vi "Pre Launch Init.vi"(11 "Child1 in":refnum<class "Child1.lvclass">) -> (0 "error out":errorcluster, 3 "Child1 out":refnum<class "Child1.lvclass">)   [LabVIEW 2020, in "Child1.lvclass"]
doc: "(<B>Filename</B>: Actor Framework.lvlib:Actor.lvclass:Pre Launch Init.vi)\n\nDefines behavior that occurs after the Launch Nested Actor method is invoked but before the actor's Actor Core method begins running.\n\nBy default, this method does nothing. A descendant class may override it to define behavior."
uses:
  Child1.lvclass
  Child1.lvclass/Child1.ctl
  <vilib>/ActorFramework/Actor/Actor.lvclass
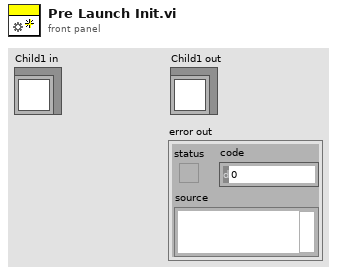
[diagram p1: front panel]
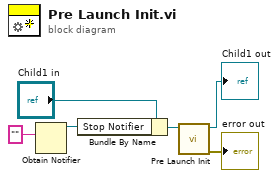
[diagram p0: block diagram]
diagram:
  n1 = Obtain Notifier(notification data type="" ("name (unnamed)")) -> (notifier out=w4:refnum<notifier>)  [unwired: 3 in, 2 out]
  n2 = Bundle By Name(cluster="Child1 in", "Stop Notifier"=w4) -> (w3:refnum<class "Child1.lvclass">)
  n3 = call-parent "Pre Launch Init.vi"("Actor in"=w3) -> ("error out"=→"error out":errorcluster, "Actor out"=→"Child1 out":refnum<class "Child1.lvclass">)  [unwired: 9 in]
